vi "random_number_led.vi"() -> ()   [LabVIEW 2025]
uses:
  <vilib>/numeric/Random Number (Range) I64.vi
  <vilib>/numeric/sub_Random U32.vi
panel:
  out "Array":i64[](array[numeric])
  out "number":i64
  out "Boolean 2":bool
  out "max value":dbl
  out "min value":dbl
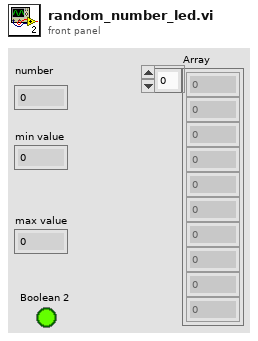
[diagram p1: front panel]
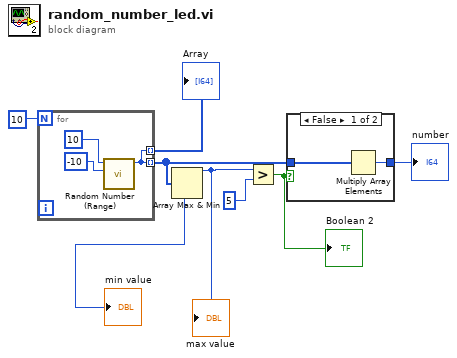
[diagram p0: block diagram]
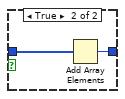
[diagram p2: hidden frame]
diagram:
  n1 = for {
    N: 10 -> [_]
    tunnel: [w9] -> w3 mode=indexing
    tunnel: [w9] -> w1 mode=indexing
    n2 = call-poly <vilib>:"Random Number (Range).vi"("lower bound (-100)"=i64 -10, "upper bound (100)"=i64 10) -> ("number"=w9:i64)  [unwired: 9 in]
  }
  "Array" <- w1
  n3 = Array Max & Min(array=w3) -> (max value=w6:i64, min value=→"min value":i64)  [unwired: 2 out]
  "max value" <- w6
  n4 = Greater?(x=w6, y=i64 5) -> (0:w4:bool)
  "Boolean 2" <- w4
  n5 = case shown="False" w4 {
    tunnel: w3 -> [w13 w15]
    tunnel: [w12 w14] -> w2
    frame False {
      n6 = Multiply Array Elements(1:w13) -> (0:w12:i64)
    }
    frame True {
      n7 = Add Array Elements(numeric array=w15) -> (sum=w14:i64)
    }
  }
  "number" <- w2
